vi "Stop Core.vi"(10 "final error code":i32, 11 "Chef State in":refnum<class "Chef State.lvclass">) -> (3 "Chef State out":refnum<class "Chef State.lvclass">)   [LabVIEW 2024, in "Chef State.lvlib" / "Chef State.lvclass"]
doc: "<p>(<strong>Filename</strong>: <span class=\"dnl\">Actor Framework.lvlib:Actor.lvclass:Stop Core.vi</span>)</p>\n<p>Defines what the actor does before it stops. Use the <strong>final error code</strong> input to determine whether the actor shut down in response to an error.</p>\n<p>By default, this method passes the Stop message along to all <a href=\"nihelplauncher://docs/csh?context=lvcore_lvcomm_af_launch_nested_actor\">auto-stop nested actors</a>. A descendant class may override this method to define additional behavior, such as shutting down any processes the actor initiated in its override of the <a href=\"nihelplauncher://docs/csh?context=lvcore_lvcomm_af_actor_core\">Actor Core</a> method.</p>"
uses:
  Chef State.lvclass
  <vilib>/ni/Actors/State Actor/State Actor/State Actor.lvclass
  Chef State.lvclass/Chef State.ctl
  <vilib>/ActorFramework/Stop Msg/Stop Msg.lvclass
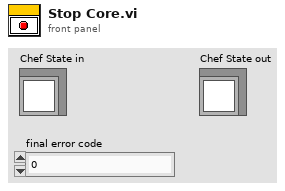
[diagram p1: front panel]
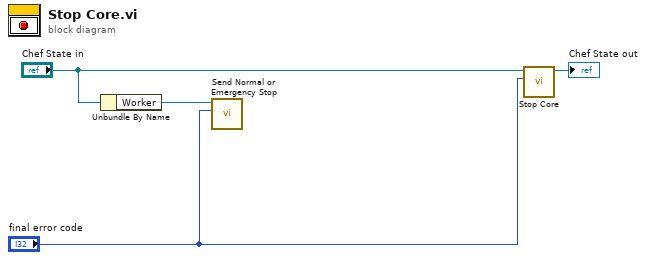
[diagram p0: block diagram]
diagram:
  n1 = Unbundle By Name("Chef State in") -> ("Worker"=w2:refnum<class "Message Enqueuer.lvclass">)
  n2 = call <vilib>:"Send Normal or Emergency Stop.vi"("final error code"="final error code", "Message Enqueuer"=w2) -> ()  [unwired: 9 in, 1 out]
  n3 = call-parent "Stop Core.vi"("final error code"="final error code", "Actor in"="Chef State in") -> ("Actor out"=→"Chef State out":refnum<class "Chef State.lvclass">)  [unwired: 9 in]
